vi "查询数据.vi"(5 "condition":string, 6 "Distinct":bool, 7 "columns":string[](array[string]), 8 "error in (no error)":errorcluster, 9 "Password":string, 10 "database":string="database1.mdb", 11 "table":string) -> (0 "error out":errorcluster, 3 "data":variant[][](array[variant]))   [LabVIEW 2016, in "数据查询.lvlib"]
uses:
  <vilib>/addons/database/Connection.llb/DB Tools Open Connec (String).vi
  <vilib>/addons/database/NI_Database_API.lvlib
  database/Access/Access Lib.lvlib
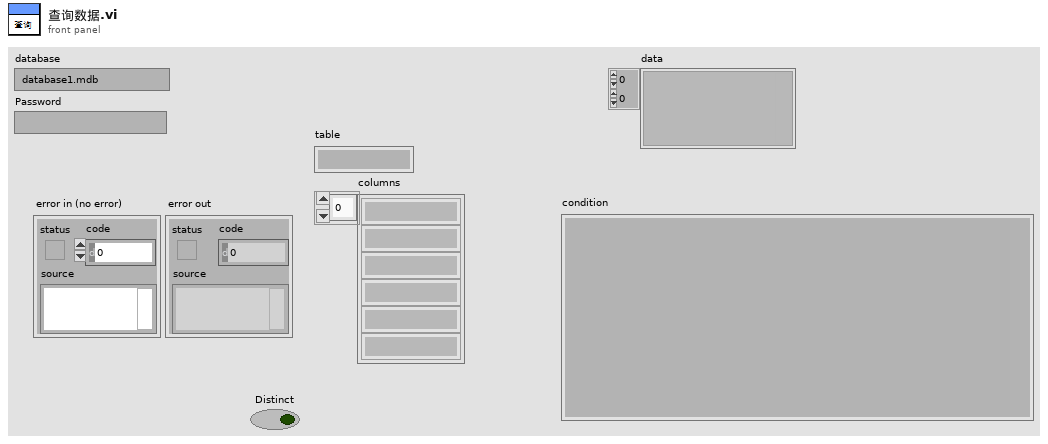
[diagram p1: front panel]
types:
  T1 = typedef "NI_Database_API.lvlib/Conn ObjectReference.ctl" = refnum<k1>
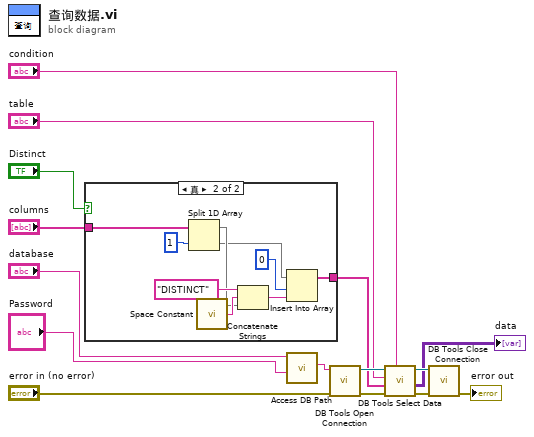
[diagram p0: block diagram]
diagram:
  n1 = case shown="真" "Distinct" {
    tunnel: "columns" -> [w16 w25]
    tunnel: [w16 w19] -> w4
    frame False {
    }
    frame True {
      n2 = Split 1D Array(array=w25, index=1 ("索引")) -> (first subarray=w18:string[], second subarray=w17:string[])
      n3 = call <vilib>:"Space Constant.vi"() -> ("String"=w22:string)
      n4 = Concatenate Strings("DISTINCT" ("字符串"), w22, w18) -> (w24:string)
      n5 = Insert Into Array(array=w17, index=0 ("索引"), new element=w24) -> (w19:string[])
    }
  }
  n6 = call "Access DB Path.vi"("Password"="Password", "database"="database") -> ("Connection information"=w2:string)  [unwired: 8 in, 1 out]
  n7 = call-poly <vilib>:"DB Tools Open Connection.vi"("error in (no error)"="error in (no error)", "connection information"=w2) -> ("error out"=w13:errorcluster, "connection reference"=w15:T1)  [unwired: 6 in]
  n8 = call <vilib>:"DB Tools Select Data.vi"("condition"="condition", "error in (no error)"=w13, "columns"=w4, "table"="table", "connection reference"=w15) -> ("error out"=w12:errorcluster, "data"=→"data":variant[][], "connection reference out"=w14:T1)  [unwired: 1 in]
  n9 = call <vilib>:"DB Tools Close Connection.vi"("error in (no error)"=w12, "connection reference"=w14) -> ("error out"=→"error out":errorcluster)  [unwired: 5 in]
